vi "check bullet collision.vi"(8 "error in (no error)":errorcluster, 11 "Game Data in":T1) -> (0 "error out":errorcluster, 3 "Game Data out":T1)   [LabVIEW 2025]
uses:
  Game Data.ctl
  Bullet Data.ctl
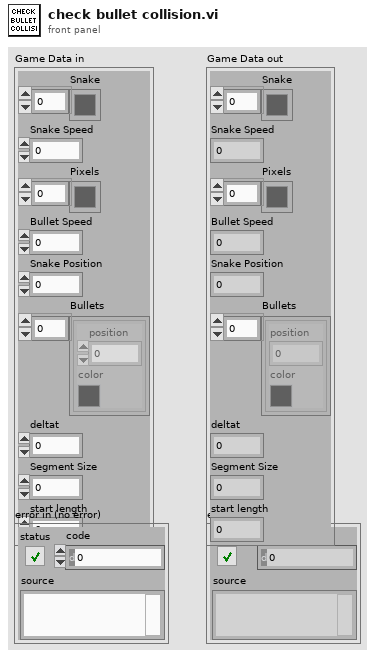
[diagram p1: front panel]
types:
  T1 = typedef "Game Data.ctl" = cluster{"Snake":u32[], "Snake Speed":dbl, "Pixels":u32[], "Bullet Speed":dbl, "Snake Position":dbl, "Bullets":T2[], "deltat":dbl, "Segment Size":dbl, "start length":u32}
  T2 = typedef "Bullet Data.ctl" = cluster{"position":dbl, "color":u32}
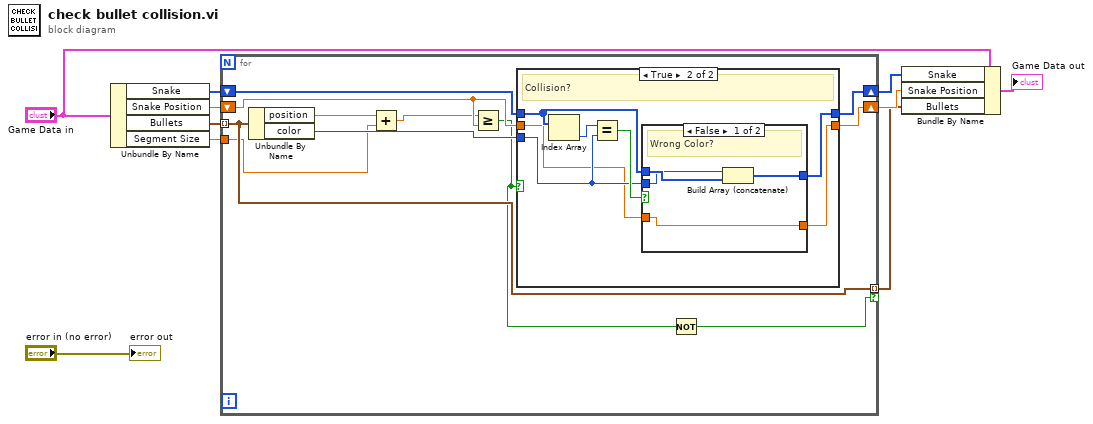
[diagram p0: block diagram]
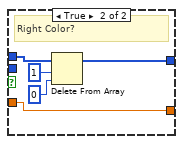
[diagram p3: hidden frame]
diagram:
  n1 = Unbundle By Name("Game Data in") -> ("Snake"=w5:u32[], "Snake Position"=w6:dbl, "Bullets"=w7:T2[], "Segment Size"=w3:dbl)
  n2 = for {
    tunnel: w7 -> [w15] mode=indexing
    shift-right: [w18] -> w4
    shift-left: w5 -> [w19]
    shift-right: [w16] -> w2
    shift-left: w6 -> [w17]
    tunnel: w3 -> [w11]
    tunnel: [w15] -> w1 mode=indexing if=w13
    n3 = Unbundle By Name(w15) -> ("position"=w21:dbl, "color"=w20:u32)
    n4 = Add(x=w21, y=w11) -> (x+y=w12:dbl)
    n5 = Greater Or Equal?(x=w12, y=w17) -> (x >= y?=w14:bool)
    n6 = case shown="True" w14 {
      tunnel: w20 -> [_ w26]
      tunnel: w19 -> [w23 w29]
      tunnel: [w23 w28] -> w18
      tunnel: w17 -> [w22 w25]
      tunnel: [w22 w24] -> w16
      frame False {
      }
      frame True {
        # "Collision?"
        n7 = Index Array(array=w29) -> (element=w30:u32)  [unwired: 1 in]
        n8 = Equal?(x=w30, y=w26) -> (x = y?=w27:bool)
        n9 = case shown="False" w27 {
          tunnel: w29 -> [w34 w39]
          tunnel: [w33 w36] -> w28
          tunnel: w26 -> [w32 _]
          tunnel: w25 -> [w31 w35]
          tunnel: [w31 w35] -> w24
          frame False {
            # "Wrong Color?"
            n10 = Build Array (concatenate)(w32, w34) -> (w33:u32[])
          }
          frame True {
            # "Right Color?"
            n11 = Delete From Array(array=w39, length=1, index=0) -> (array with subset deleted=w36:u32[])  [unwired: 1 out]
          }
        }
      }
    }
    n12 = Not(x=w14) -> (.not. x?=w13:bool)
  }
  n13 = Bundle By Name(cluster="Game Data in", "Snake"=w4, "Snake Position"=w2, "Bullets"=w1) -> (→"Game Data out":T1)
  "error out" <- "error in (no error)"
